vi "Configure Modulation (Pulse).vi"(0 "VISA resource name":refnum<visa-resource-name>, 1 "Enable Pulse Modulation (T:Enable)":bool=TRUE, 2 "Pulse Modulation Source (1: Internal Free-Run)":u16(ring)=1 items=["Internal Square", "Internal Free-Run", "Internal Triggered", "Internal Adjustable Doublet", "Internal Doublet", "Internal Gated", "External Pulse", "Scalar"], 3 "Pulse Rate (400 Hz)":dbl=400.0, 5 "Pulse Delay1 (0 s)":dbl, 7 "Pulse Delay2 (0 s)":dbl, 9 "Pulse Period (4 us)":dbl=4e-06, 11 "error in (no error)":errorcluster, 12 "Pulse Width1 (1 us)":dbl=1e-06, 13 "Pulse Width2 (2 us)":dbl=2e-06, 14 "External Polarity (0: Normal)":u16(ring) items=["Normal", "Inverted"]) -> (4 "VISA resource name out":refnum<visa-resource-name>, 15 "error out":errorcluster)   [LabVIEW 2009, in "Agilent PSG MXG Series.lvlib"]
doc: "Configures pulse modulation.\n\n<B>Notes:</B>\n(1) This VI is <B>NOT</B> valid in E8247C.\n\n(2) For N5181A, N5182A, N5183A, this VI is valid only when the instrument installs <B>Option UNU</B> (Pulse modulation) and <B>Option UNW</B> (Narrow pulse modulation).\n\n(3) For E8257D, E8267D, this VI is valid only when the instrument installs <B>Option UNU</B> or <B>Option UNW</B>."
uses:
  Agilent PSG MXG Series.lvlib
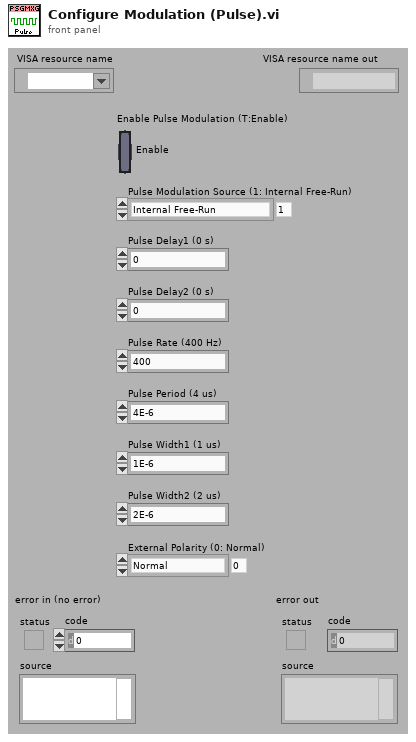
[diagram p1: front panel]
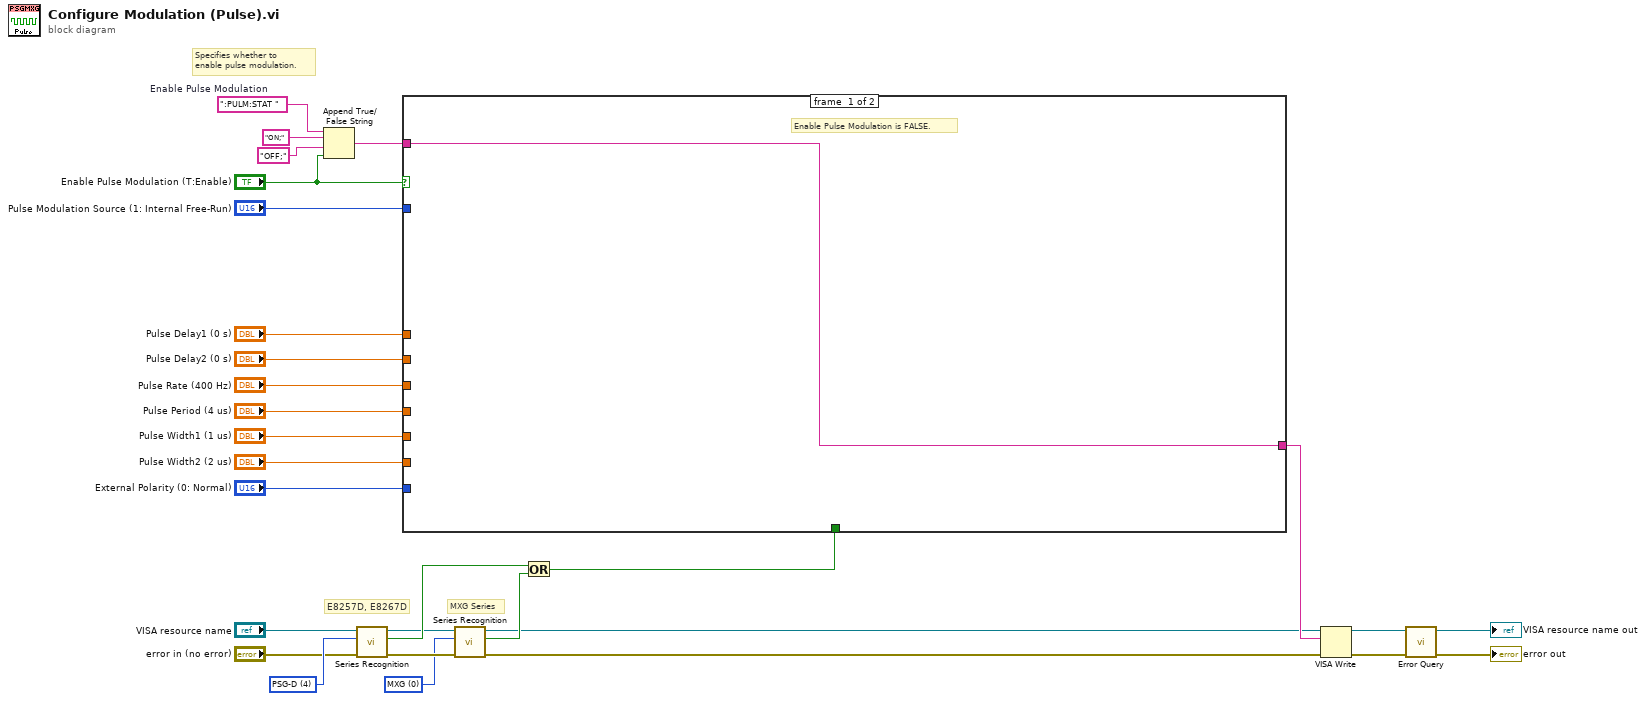
[diagram p0: block diagram]
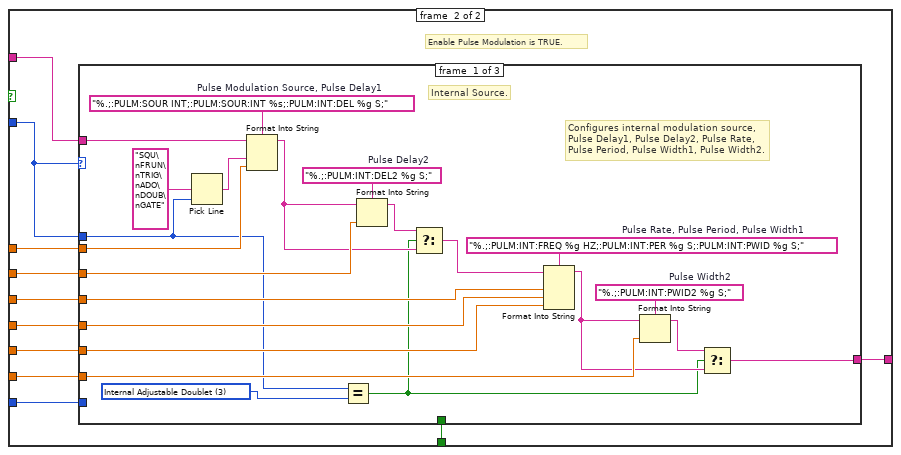
[diagram p2: hidden frame]
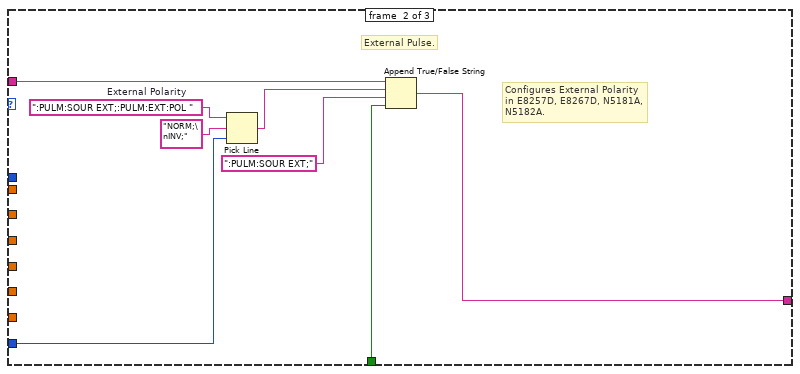
[diagram p3: hidden frame]
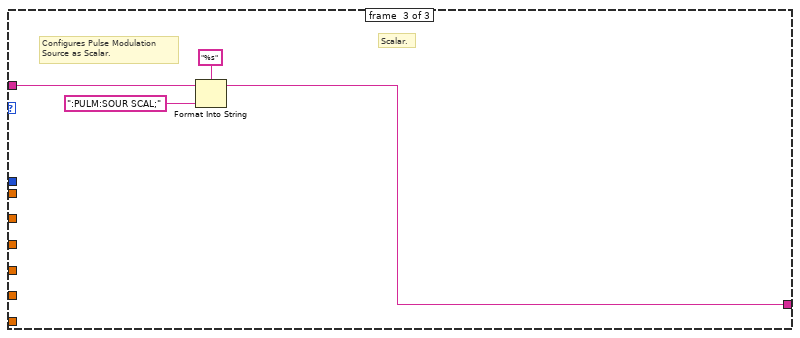
[diagram p4: hidden frame]
diagram:
  w8 = u16 0 items=["MXG", "PSG", "PSG-A", "PSG-C", "PSG-D"] ("Series Type (0: MXG)")
  w12 = u16 4 items=["MXG", "PSG", "PSG-A", "PSG-C", "PSG-D"] ("Series Type (0: MXG)")
  w29 = ":PULM:STAT "  # Enable Pulse Modulation
  # "Specifies whether to\nenable pulse modulation."
  # "E8257D, E8267D"
  # "MXG Series"
  n1 = Append True/False String(1:"Enable Pulse Modulation (T:Enable)", 2:"OFF;" ("false string"), 3:"ON;" ("true string"), 4:w29) -> (0:w24:string)
  n2 = call "Series Recognition.vi"("error in (no error)"="error in (no error)", "Series Type (0: MXG)"=w12, "VISA resource name"="VISA resource name") -> ("error out"=w9:errorcluster, "Is Series Correct"=w11:bool, "VISA resource name out"=w10:refnum<visa-resource-name>)  [unwired: 6 out]
  n3 = call "Series Recognition.vi"("error in (no error)"=w9, "Series Type (0: MXG)"=w8, "VISA resource name"=w10) -> ("error out"=w5:errorcluster, "Is Series Correct"=w7:bool, "VISA resource name out"=w6:refnum<visa-resource-name>)  [unwired: 6 out]
  n4 = Or(x=w11, y=w7) -> (x .or. y?=w13:bool)
  n5 = case shown="True" "Enable Pulse Modulation (T:Enable)" {
    tunnel: "Pulse Modulation Source (1: Internal Free-Run)" -> [_ w32]
    tunnel: w24 -> [w30 w41]
    tunnel: "Pulse Delay1 (0 s)" -> [_ w40]
    tunnel: "Pulse Delay2 (0 s)" -> [_ w39]
    tunnel: "Pulse Rate (400 Hz)" -> [_ w38]
    tunnel: "Pulse Period (4 us)" -> [_ w37]
    tunnel: "Pulse Width1 (1 us)" -> [_ w36]
    tunnel: "Pulse Width2 (2 us)" -> [_ w35]
    tunnel: "External Polarity (0: Normal)" -> [_ w34]
    tunnel: [w30 w33] -> w16
    tunnel: w13 -> [_ w31]
    frame #0 {
      # "Enable Pulse Modulation is FALSE."
    }
    frame #1 {
      # "Enable Pulse Modulation is TRUE."
      n6 = case shown="0, Default" w32 {
        tunnel: w32 -> [w43 _ _]
        tunnel: w41 -> [w59 w66 w75]
        tunnel: w40 -> [w58 _ _]
        tunnel: w39 -> [w57 _ _]
        tunnel: w38 -> [w52 _ _]
        tunnel: w37 -> [w51 _ _]
        tunnel: w36 -> [w49 _ _]
        tunnel: w35 -> [w48 _ _]
        tunnel: w34 -> [_ w69 _]
        tunnel: [w45 w65 w72] -> w33
        tunnel: w31 -> [_ w64 _]
        frame #0 {
          w44 = u16 3 items=["Internal Square", "Internal Free-Run", "Internal Triggered", "Internal Adjustable Doublet", "Internal Doublet", "Internal Gated", "External Pulse", "Scalar"] ("Pulse Modulation Source (1: Internal Free-Run)")
          w50 = "%.;:PULM:INT:PWID2 %g S;"  # Pulse Width2
          w53 = "%.;:PULM:INT:FREQ %g HZ;:PULM:INT:PER %g S;:PULM:INT:PWID %g S;"  # Pulse Rate, Pulse Period, Pulse Width1
          w60 = "%.;:PULM:SOUR INT;:PULM:SOUR:INT %s;:PULM:INT:DEL %g S;"  # Pulse Modulation Source, Pulse Delay1
          w61 = "%.;:PULM:INT:DEL2 %g S;"  # Pulse Delay2
          # "Configures internal modulation source,\nPulse Delay1, Pulse Delay2, Pulse Rate,\nPulse Period, Pulse Width1, Pulse Width2."
          # "Internal Source."
          n7 = Pick Line(multi-line string="SQU\nFRUN\nTRIG\nADO\nDOUB\nGATE", line index=w43) -> (output string=w62:string)  [unwired: 1 out]
          n8 = Format Into String(format string=w60, initial string=w59, w62, w58) -> (resulting string=w55:string)  [unwired: 1 in, 1 out]
          n9 = Equal?(x=w43, y=w44) -> (x = y?=w42:bool)
          n10 = Format Into String(format string=w61, initial string=w55, w57) -> (resulting string=w56:string)  [unwired: 1 in, 1 out]
          n11 = Select(t=w56, s=w42, f=w55) -> (s? t:f=w54:string)
          n12 = Format Into String(format string=w53, initial string=w54, w52, w51, w49) -> (resulting string=w46:string)  [unwired: 1 in, 1 out]
          n13 = Format Into String(format string=w50, initial string=w46, w48) -> (resulting string=w47:string)  [unwired: 1 in, 1 out]
          n14 = Select(t=w47, s=w42, f=w46) -> (s? t:f=w45:string)
        }
        frame #1 {
          w71 = ":PULM:SOUR EXT;:PULM:EXT:POL "  # External Polarity
          # "Configures External Polarity\nin E8257D, E8267D, N5181A,\nN5182A."
          # "External Pulse."
          n15 = Pick Line(string ("")=w71, multi-line string="NORM;\nINV;", line index=w69) -> (output string=w68:string)
          n16 = Append True/False String(1:w64, 2:":PULM:SOUR EXT;" ("false string"), 3:w68, 4:w66) -> (0:w65:string)
        }
        frame #2 {
          # "Configures Pulse Modulation\nSource as Scalar."
          # "Scalar."
          n17 = Format Into String(format string="%s", initial string=w75, ":PULM:SOUR SCAL;" ("true string")) -> (resulting string=w72:string)  [unwired: 1 in, 1 out]
        }
      }
    }
  }
  n18 = VISA Write(VISA resource name=w6, write buffer=w16, error in (no error)=w5) -> (VISA resource name out=w15:refnum<visa-resource-name>, error out=w14:errorcluster)  [unwired: 1 out]
  n19 = call "Error Query.vi"("error in (no error)"=w14, "VISA resource name"=w15) -> ("error out"=→"error out":errorcluster, "VISA resource name out"=→"VISA resource name out":refnum<visa-resource-name>)  [unwired: 8 out]
